vi "FGV_ActorTest_Class.vi"(0 "Action":T2(ring), 5 "Actor Test":refnum<class "Actor Test (Default).lvclass">, 7 "Actor class":string, 9 "Group Name":string, 11 "error in (no error)":errorcluster, 12 "Parameter (Json) en entrée":string) -> (4 "Actor Test":refnum<class "Actor Test (Default).lvclass">, 6 "List Test":T1(array[cluster]), 14 "Parameter (Json) en sortie":string, 15 "error out":errorcluster)   [LabVIEW 2020, in "Library Commun.lvlib"]
uses:
  Library Commun.lvlib
  Class/Sequencer/Actor Test (Default)/Actor Test (Default).lvclass
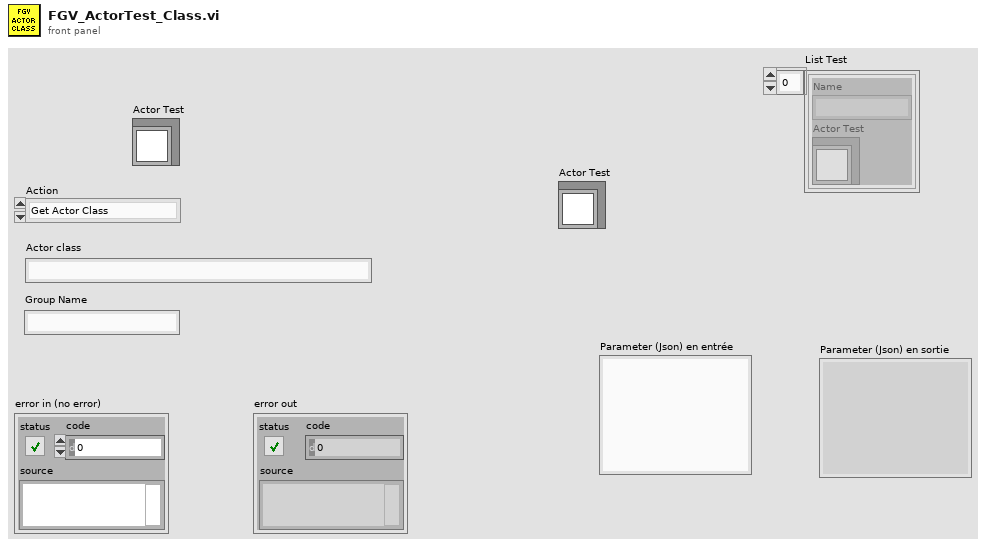
[diagram p1: front panel]
types:
  T1 = cluster{"Name":string, "Actor Test":refnum<class "Actor Test (Default).lvclass">}[]
  T2 = enum16{"Get Actor Class", "Set Actor object", "Get Actor object", "List Actor", "Init"}
  T3 = cluster{"Group Name":string, "Actor Test":refnum<class "Actor Test (Default).lvclass">}
  T4 = cluster{"Group Name":string, "Actor Test":refnum<class "Actor Test (Default).lvclass">}[]
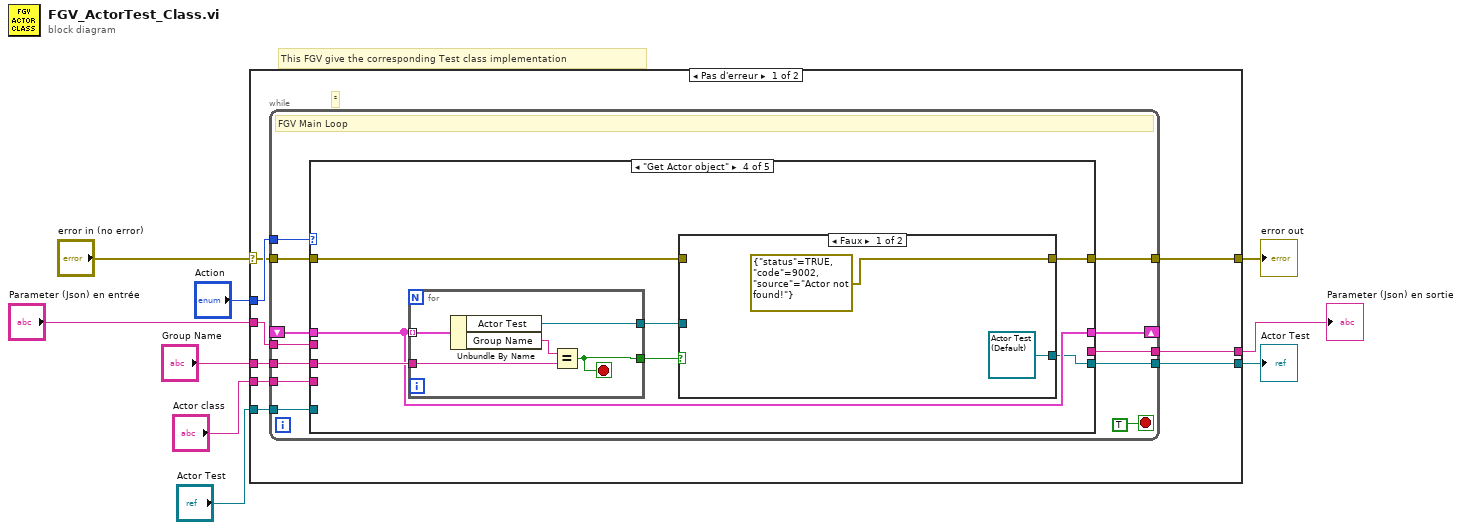
[diagram p0: block diagram]
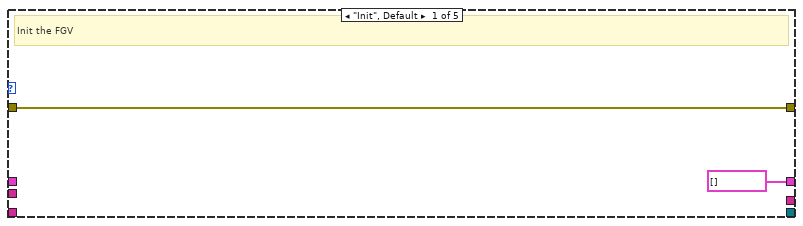
[diagram p2: hidden frame]
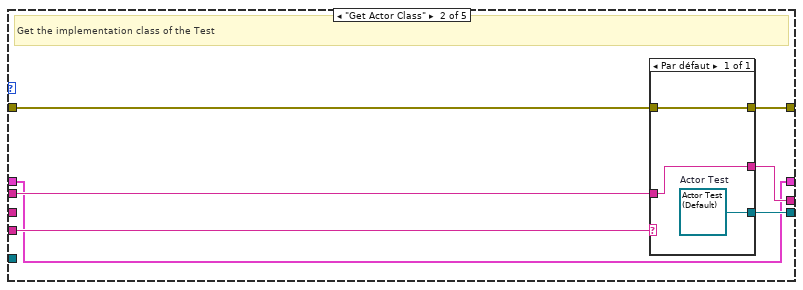
[diagram p3: hidden frame]
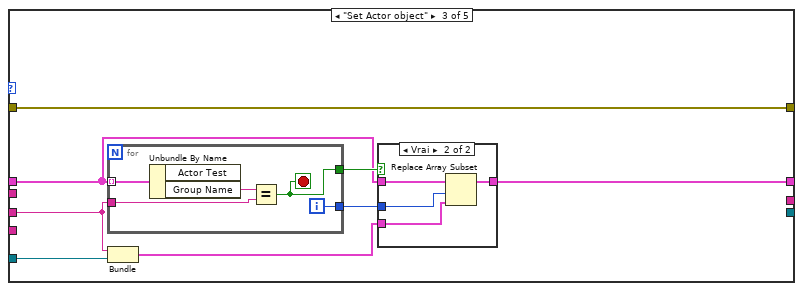
[diagram p4: hidden frame]
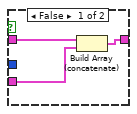
[diagram p5: hidden frame]
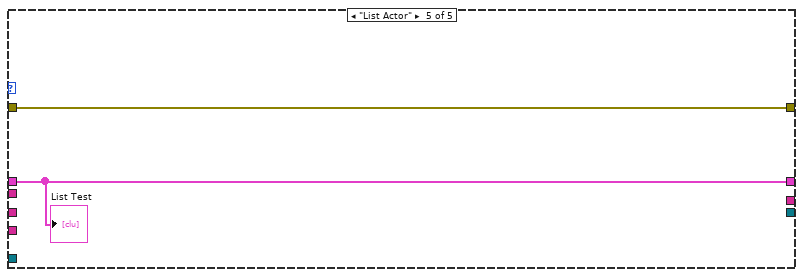
[diagram p7: hidden frame]
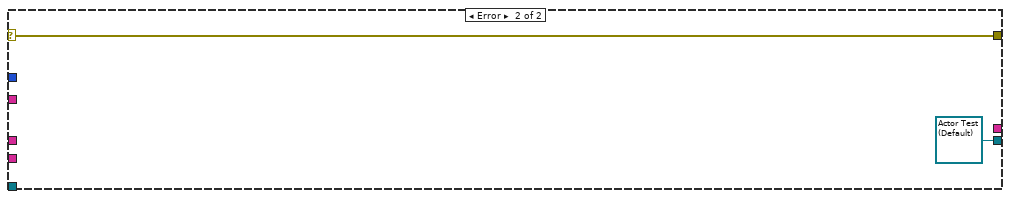
[diagram p8: hidden frame]
diagram:
  # "This FGV give the corresponding Test class implementation"
  n1 = case shown="Pas d'erreur" "error in (no error)" {
    selector: "error in (no error)" -> [w17 w82]
    tunnel: [w16 w82] -> w8
    tunnel: "Action" -> [w18 _]
    tunnel: "Actor class" -> [w15 _]
    tunnel: [w14 refnum<class "Actor Test (Default).lvclass"> refnum ("Actor Test 2")] -> w5
    tunnel: [w13 _] -> w4
    tunnel: "Parameter (Json) en entrée" -> [w12 _]
    tunnel: "Actor Test" -> [w11 _]
    tunnel: "Group Name" -> [w10 _]
    frame No Error {
      # "²"
      n2 = while {
        tunnel: w18 -> [w30]
        tunnel: w17 -> [w29]
        tunnel: [w28] -> w16
        tunnel: w15 -> [w27]
        tunnel: [w25] -> w14
        tunnel: [w24] -> w13
        tunnel: w12 -> [w23]
        shift-right: [w22] -> _
        shift-left: _ -> [w21]
        tunnel: w11 -> [w20]
        tunnel: w10 -> [w19]
        stop <- TRUE stop-if-true
        # "FGV Main Loop"
        n3 = case shown="\"Get Actor object\"" w30 {
          tunnel: w29 -> [w32 w37 w50 w64 w79]
          tunnel: [w32 w36 w50 w63 w79] -> w28
          tunnel: w27 -> [_ w39 _ _ _]
          tunnel: [_ w38 _ w65 _] -> w25
          tunnel: [_ w35 _ _ _] -> w24
          tunnel: w23 -> [_ w34 _ _ _]
          tunnel: [T1 [] ("List Test") w33 w46 w68 w80] -> w22
          tunnel: w21 -> [_ w33 w47 w68 w80]
          tunnel: w20 -> [_ _ w45 _ _]
          tunnel: w19 -> [_ _ w44 w69 _]
          frame "Init", Default {
            # "Init the FGV"
          }
          frame "Get Actor Class" {
            # "Get the implementation class of the Test"
            n4 = case shown="Par défaut" w39 {
              tunnel: [w40] -> w38
              tunnel: w37 -> [w41]
              tunnel: [w41] -> w36
              tunnel: [w42] -> w35
              tunnel: w34 -> [w42]
              frame Par défaut {
                w40 = refnum<class "Actor Test (Default).lvclass"> refnum  # Actor Test
              }
            }
          }
          frame "Set Actor object" {
            n5 = for {
              tunnel: w47 -> [w62] mode=indexing
              tunnel: [w60] -> w49
              tunnel: [w59] -> w48
              tunnel: w44 -> [w58]
              i -> [w59]
              stop <- w60 stop-if-true
              n6 = Unbundle By Name(w62) -> ("Group Name"=w61:string)  [unwired: 1 out]
              n7 = Equal?(x=w61, y=w58) -> (x = y?=w60:bool)
            }
            n8 = Bundle("Group Name"=w44, "Actor Test"=w45) -> (w43:T3)  [unwired: 1 in]
            n9 = case shown="Vrai" w49 {
              tunnel: [w53 w54] -> w46
              tunnel: w47 -> [w52 w57]
              tunnel: w43 -> [w51 w55]
              tunnel: w48 -> [_ w56]
              frame False {
                n10 = Build Array (concatenate)(w52, w51) -> (w53:T4)
              }
              frame True {
                n11 = Replace Array Subset(array=w57, new element=w55, index=w56) -> (w54:T4)
              }
            }
          }
          frame "Get Actor object" {
            n12 = for {
              tunnel: w68 -> [w78] mode=indexing
              tunnel: w69 -> [w76]
              tunnel: [w75] -> w66
              tunnel: [w74] -> w67
              stop <- w74 stop-if-true
              n13 = Unbundle By Name(w78) -> ("Actor Test"=w75:refnum<class "Actor Test (Default).lvclass">, "Group Name"=w77:string)
              n14 = Equal?(x=w77, y=w76) -> (x = y?=w74:bool)
            }
            n15 = case shown="Faux" w67 {
              tunnel: [refnum<class "Actor Test (Default).lvclass"> refnum ("Actor Test") w73] -> w65
              tunnel: w66 -> [_ w73]
              tunnel: w64 -> [_ w72]
              tunnel: [errorcluster {"status"=TRUE, "code"=9002, "source"="Actor not found!"} ("error constant") w72] -> w63
              frame False {
              }
              frame True {
              }
            }
          }
          frame "List Actor" {
            "List Test" <- w80
          }
        }
      }
    }
    frame Error {
    }
  }
  "error out" <- w8
  "Actor Test" <- w5
  "Parameter (Json) en sortie" <- w4
